vi "Unit Test SWIR.vi"() -> ()   [LabVIEW 2018]
uses:
  PPLs/Camera/Parent/Camera.lvlibp/Custom Controls/Camera Setting.ctl
  Custom Controls/enm_States.ctl
  PPLs/Camera/Parent/Camera.lvlibp/1abvi3w/vi.lib/vision/Image Controls.llb/IMAQ Image.ctl
  PPLs/Camera/Parent/Camera.lvlibp/Camera.lvclass
  Bobcat 640.lvclass
  PPLs/Camera/Parent/Camera.lvlibp
panel:
  in  "PPLs Folder Path":path=path "C:/AME Test Engineering/LabVIEW/PPLs"
  in  "INI File Path":path
  in  "Value":string
  in  "Setting":T1
  in  "Update Setting":bool
  in  "Config_Setting":string(combo)
  in  "Set Calibration":bool
  in  "Stop":bool
  in  "Grab":bool
  out "Connected?":bool
  in  "Error In":errorcluster
  out "Error Out":errorcluster
  in  "Snap":bool
  out "Image Display":T2(plugin-control)
  in  "Device":string="Camera"
  # "Image Acquisition"
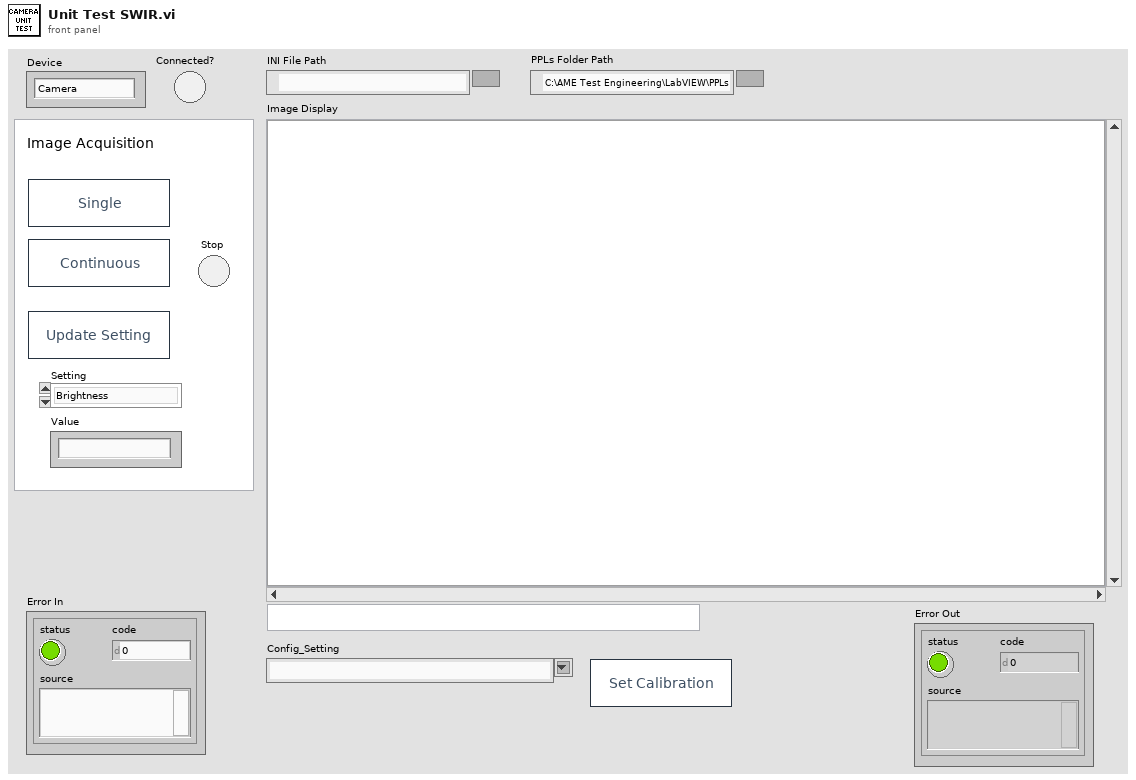
[diagram p1: front panel]
types:
  T1 = typedef "Camera.lvlibp/Camera.lvclass/Camera Setting.ctl" = enum16{"Brightness", "Rotation", "Contrast", "Exposure", "Frame Rate", "Gain", "Gamma", "Image Resolution", "Sharpness"}
  T2 = typedef "IMAQ Image.ctl" = refnum<image>
  T3 = typedef "Bobcat 640.lvlib/Bobcat 640.lvclass/enm_States.ctl" = enum16{"Wait for Event", "Snap", "Grab", "Exit"}
  T4 = typedef "Camera.lvlibp/IMAQ Image.ctl" = refnum<image>
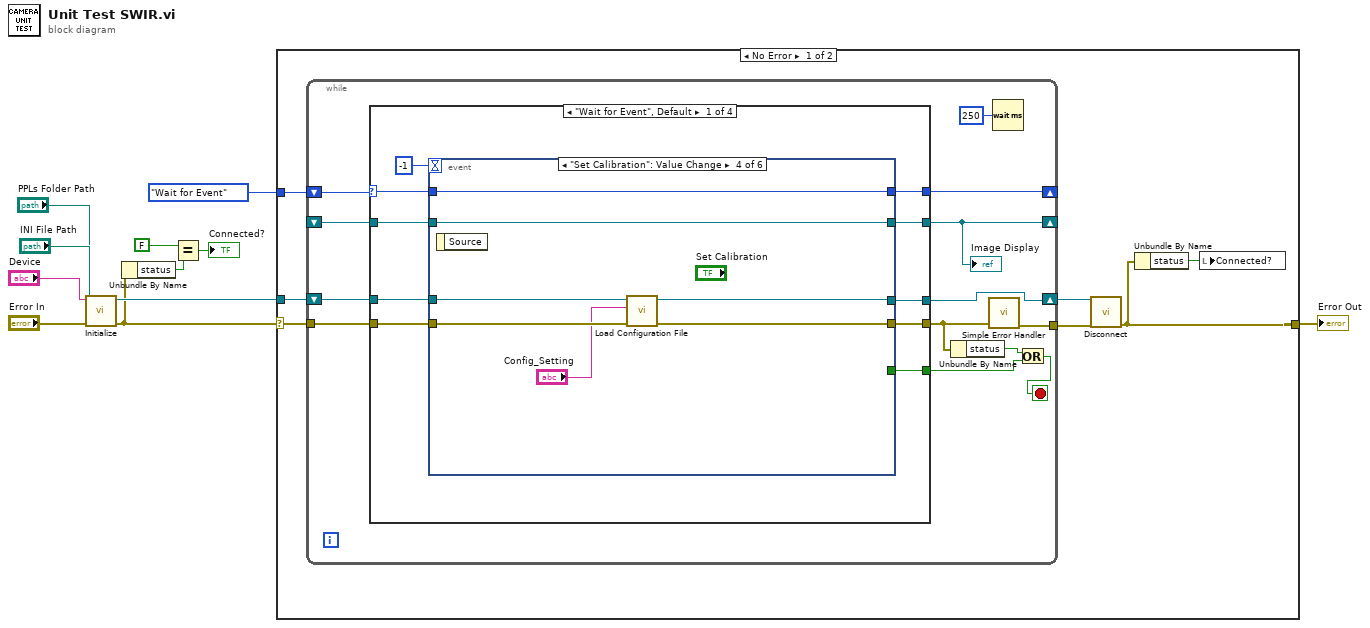
[diagram p0: block diagram]
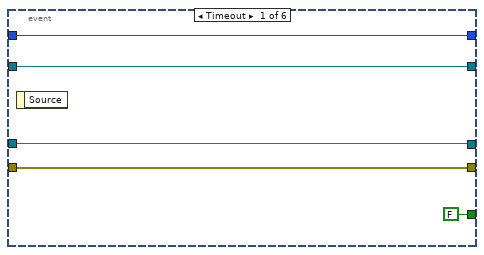
[diagram p2: hidden frame]
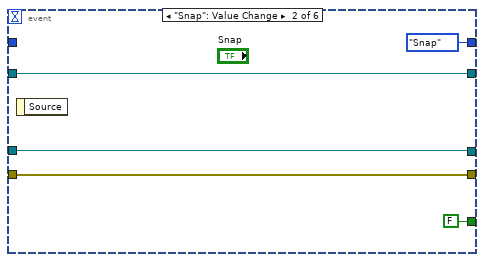
[diagram p3: hidden frame]
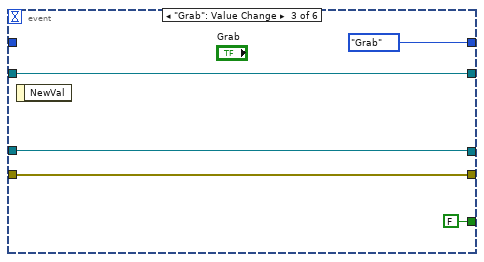
[diagram p4: hidden frame]
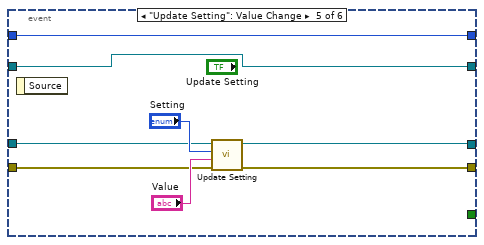
[diagram p5: hidden frame]
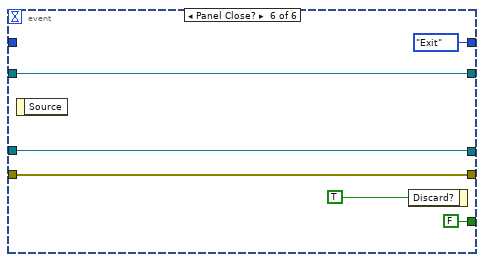
[diagram p6: hidden frame]
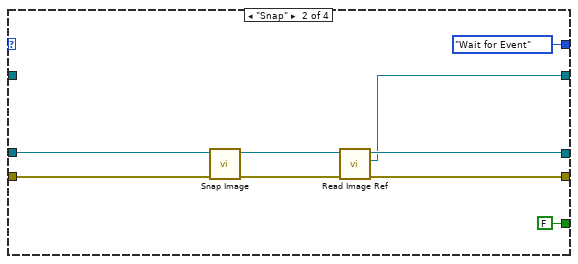
[diagram p7: hidden frame]
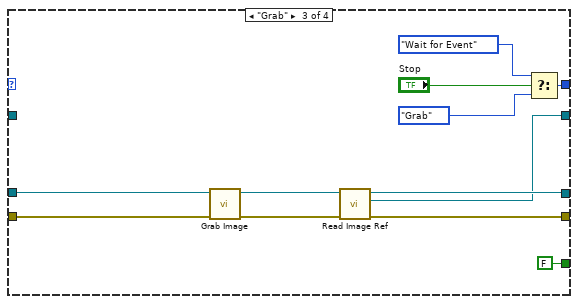
[diagram p8: hidden frame]
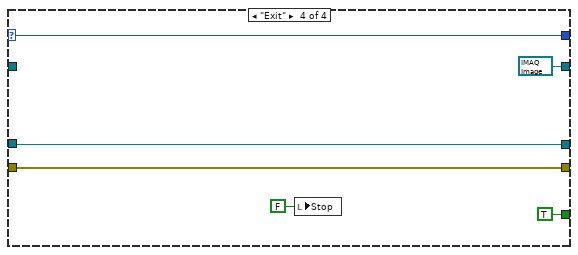
[diagram p9: hidden frame]
diagram:
  n1 = call "Initialize.vi"("error in"="Error In", "PPLs Folder Path"="PPLs Folder Path", "INI File Path"="INI File Path", "Device"="Device") -> ("error out"=w6:errorcluster, "Camera out"=w11:refnum<class "Camera.lvclass">)  [unwired: 6 in]
  n2 = Unbundle By Name(w6) -> ("status"=w5:bool)
  n3 = Equal?(x=FALSE, y=w5) -> (x = y?=→"Connected?":bool)
  n4 = case shown="No Error" w6 {
    selector: w6 -> [w17 w105]
    tunnel: w11 -> [w18 _]
    tunnel: [w14 w105] -> w9
    tunnel: enm_States."Wait for Event" -> [w12 _]
    frame No Error {
      n5 = while {
        shift-right: [w29] -> w15
        shift-left: w18 -> [w31]
        tunnel: w17 -> [w30]
        tunnel: [w28] -> w16
        shift-right: [w26] -> _
        shift-left: _ -> [w27]
        shift-right: [w24] -> _
        shift-left: w12 -> [w25]
        stop <- w19 stop-if-true
        n6 = case shown="\"Wait for Event\", Default" w25 {
          selector: w25 -> [w32 _ _ w104]
          tunnel: w31 -> [w41 w85 w98 w101]
          tunnel: w30 -> [w40 w84 w97 w100]
          tunnel: [w39 w80 w93 w101] -> w29
          tunnel: [w38 w81 w94 w100] -> w22
          tunnel: [w36 FALSE ("Discard?") FALSE ("Discard?") TRUE ("Discard?")] -> w20
          tunnel: w27 -> [w35 _ _ _]
          tunnel: [w34 w79 w92 T4 refnum ("Image")] -> w26
          tunnel: [w33 enm_States."Wait for Event" w87 w104] -> w24
          frame "Wait for Event", Default {
            n7 = event shown="[3] \"Set Calibration\": Value Change" {
              selector: _ -> [_ _ _ _ _ _]
              dyn-events: _ -> [_ _ _ _ _ _]
              timeout: -1 -> [_ _ _ _ _ _]
              tunnel: w41 -> [w46 w50 w56 w62 w68 w76]
              tunnel: w40 -> [w45 w51 w55 w60 w64 w75]
              tunnel: [w46 w50 w56 w61 w67 w76] -> w39
              tunnel: [w45 w51 w55 w59 w65 w75] -> w38
              tunnel: [FALSE ("Discard?") FALSE ("Discard?") FALSE ("Discard?") _ _ FALSE ("Discard?")] -> w36
              tunnel: [w44 w48 w53 w57 w66 w74] -> w34
              tunnel: w35 -> [w44 w48 w53 w57 w66 w74]
              tunnel: [w43 enm_States."Snap" enm_States."Grab" w63 w71 enm_States."Exit"] -> w33
              tunnel: w32 -> [w43 _ _ w63 w71 _]
              event Timeout {
                n8 = event-data() -> ()  [unwired: 1 in, 1 out]
              }
              event "Snap": Value Change {
                n9 = event-data() -> ()  [unwired: 1 in, 1 out]
              }
              event "Grab": Value Change {
                n10 = event-data() -> ()  [unwired: 1 in, 1 out]
              }
              event "Set Calibration": Value Change {
                n11 = event-data() -> ()  [unwired: 1 in, 1 out]
                n12 = call-dynamic "Load Configuration File.vi"("error in"=w60, "Filename"="Config_Setting", "Camera in"=w62) -> ("error out"=w59:errorcluster, "Camera out"=w61:refnum<class "Camera.lvclass">)  [unwired: 6 in, 1 out]
              }
              event "Update Setting": Value Change {
                n13 = event-data() -> ()  [unwired: 1 in, 1 out]
                n14 = call-dynamic "Update Setting.vi"("Camera in"=w68, "Setting"="Setting", "Value"="Value", "error in"=w64) -> ("Camera out"=w67:refnum<class "Camera.lvclass">, "error out"=w65:errorcluster)  [unwired: 4 in, 1 out]
              }
              event Panel Close? {
                n15 = event-data() -> ()  [unwired: 1 in, 1 out]
                n16 = event-data("Discard?"=TRUE) -> ()  [unwired: 1 in, 1 out]
              }
            }
          }
          frame "Snap" {
            n17 = call-dynamic "Snap Image.vi"("error in (no error)"=w84, "Camera in"=w85) -> ("error out"=w82:errorcluster, "Camera out"=w83:refnum<class "Camera.lvclass">)  [unwired: 8 in]
            n18 = call "Read Image Ref.vi"("error in (no error)"=w82, "Camera in"=w83) -> ("error out"=w81:errorcluster, "Image"=w79:T4, "Camera out"=w80:refnum<class "Camera.lvclass">)  [unwired: 7 in]
          }
          frame "Grab" {
            n19 = call-dynamic "Grab Image.vi"("error in (no error)"=w97, "Camera in"=w98) -> ("error out"=w95:errorcluster, "Camera out"=w96:refnum<class "Camera.lvclass">)  [unwired: 8 in]
            n20 = call "Read Image Ref.vi"("error in (no error)"=w95, "Camera in"=w96) -> ("error out"=w94:errorcluster, "Image"=w92:T4, "Camera out"=w93:refnum<class "Camera.lvclass">)  [unwired: 7 in]
            n21 = Select(t=enm_States."Wait for Event", s="Stop", f=enm_States."Grab") -> (s? t:f=w87:T3)
          }
          frame "Exit" {
            n22 = local write "Stop"(FALSE ("Stop")) -> ()
          }
        }
        "Image Display" <- w26
        n23 = Unbundle By Name(w22) -> ("status"=w21:bool)
        n24 = call <vilib>:"Simple Error Handler.vi"("error in (no error)"=w22) -> ("error out"=w28:errorcluster)  [unwired: 4 in, 4 out]
        n25 = Wait (ms)(milliseconds to wait=u32 250) -> ()  [unwired: 1 out]
        n26 = Or(x=w21, y=w20) -> (x .or. y?=w19:bool)
      }
      n27 = call-dynamic "Disconnect.vi"("error in (no error)"=w16, "Camera in"=w15) -> ("error out"=w14:errorcluster)  [unwired: 8 in, 1 out]
      n28 = Unbundle By Name(w14) -> ("status"=w13:bool)
      n29 = local write "Connected?"(w13) -> ()
    }
    frame Error {
    }
  }
  "Error Out" <- w9
